vi "Digital Input 16-32.vi"(9 "S.no":string[](array[string]), 10 "Sting Array":string[](array[string]), 11 "Digital In _DAQ":bool[](array[boolean])) -> (2 "array":T1(array[cluster]))   [LabVIEW 2015]
panel:
  in  "output cluster":T2
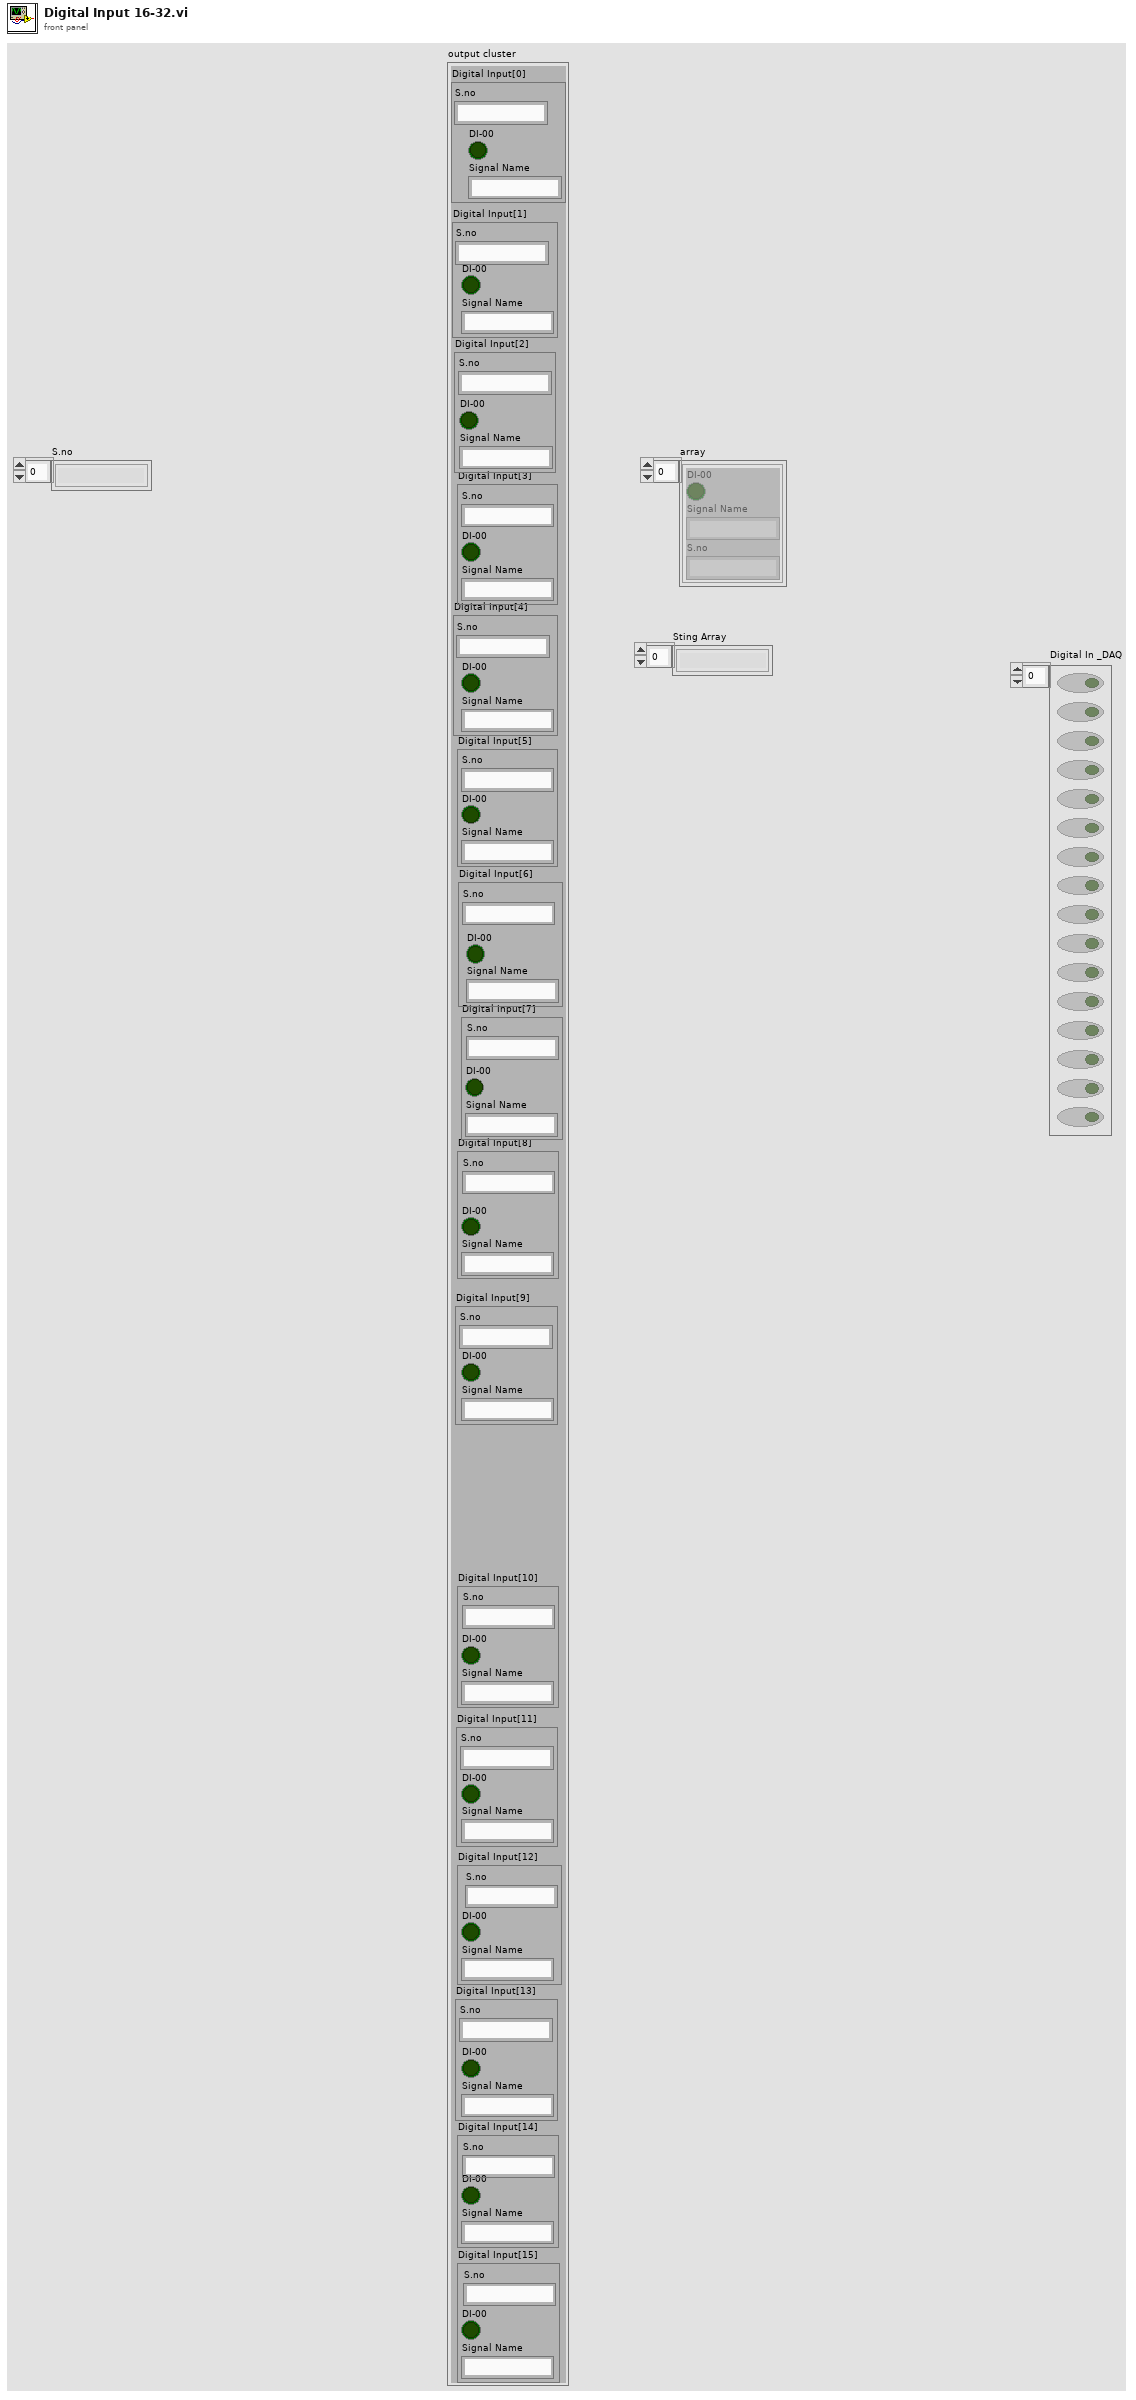
[diagram p1: front panel]
types:
  T1 = cluster{"DI-00":bool, "Signal Name":string, "S.no":string}[]
  T2 = cluster{"Digital Input[0]":cluster{"DI-00":bool, "Signal Name":string, "S.no":string}, "Digital Input[1]":cluster{"DI-00":bool, "Signal Name":string, "S.no":string}, "Digital Input[2]":cluster{"DI-00":bool, "Signal Name":string, "S.no":string}, "Digital Input[3]":cluster{"DI-00":bool, "Signal Name":string, "S.no":string}, "Digital Input[4]":cluster{"DI-00":bool, "Signal Name":string, "S.no":string}, "Digital Input[5]":cluster{"DI-00":bool, "Signal Name":string, "S.no":string}, "Digital Input[6]":cluster{"DI-00":bool, "Signal Name":string, "S.no":string}, "Digital Input[7]":cluster{"DI-00":bool, "Signal Name":string, "S.no":string}, "Digital Input[8]":cluster{"DI-00":bool, "Signal Name":string, "S.no":string}, "Digital Input[9]":cluster{"DI-00":bool, "Signal Name":string, "S.no":string}, "Digital Input[10]":cluster{"DI-00":bool, "Signal Name":string, "S.no":string}, "Digital Input[11]":cluster{"DI-00":bool, "Signal Name":string, "S.no":string}, "Digital Input[12]":cluster{"DI-00":bool, "Signal Name":string, "S.no":string}, "Digital Input[13]":cluster{"DI-00":bool, "Signal Name":string, "S.no":string}, "Digital Input[14]":cluster{"DI-00":bool, "Signal Name":string, "S.no":string}, "Digital Input[15]":cluster{"DI-00":bool, "Signal Name":string, "S.no":string}}
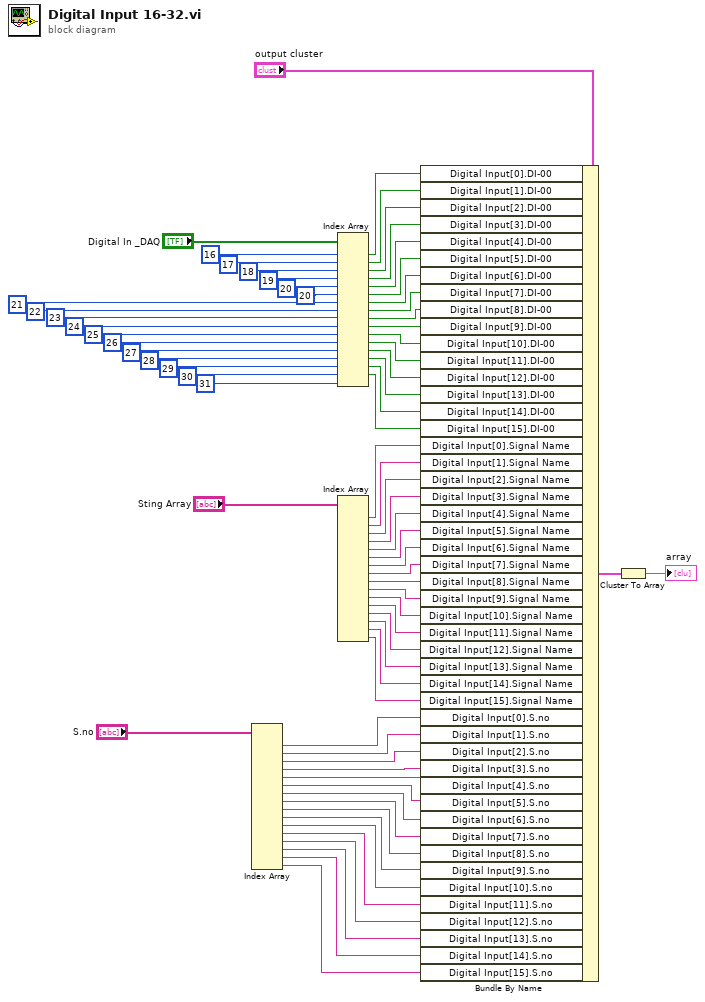
[diagram p0: block diagram]
diagram:
  n1 = Index Array(array="S.no") -> (element #1=w34:string, element #2=w32:string, element #3=w31:string, element #4=w30:string, element #5=w29:string, element #6=w28:string, element #7=w27:string, element #8=w26:string, element #9=w25:string, element #10=w24:string, element #11=w23:string, element #12=w22:string, element #13=w21:string, element #14=w20:string, element #15=w19:string, element #16=w18:string)  [unwired: 16 in]
  n2 = Index Array(array="Digital In _DAQ", index #1=16 ("index"), index #2=17 ("index"), index #3=18 ("index"), index #4=19 ("index"), index #5=20 ("index"), index #6=20 ("index"), index #7=21 ("index"), index #8=22 ("index"), index #9=23 ("index"), index #10=24 ("index"), index #11=25 ("index"), index #12=26 ("index"), index #13=27 ("index"), index #14=28 ("index"), index #15=29 ("index"), index #16=30 ("index"), index #17=31 ("index")) -> (element #1=w71:bool, element #2=w70:bool, element #3=w69:bool, element #4=w68:bool, element #5=w67:bool, element #6=w66:bool, element #7=w65:bool, element #8=w64:bool, element #9=w63:bool, element #10=w62:bool, element #11=w61:bool, element #12=w60:bool, element #13=w59:bool, element #14=w58:bool, element #15=w57:bool, element #16=w56:bool)  [unwired: 1 out]
  n3 = Index Array(array="Sting Array") -> (element #1=w54:string, element #2=w53:string, element #3=w52:string, element #4=w51:string, element #5=w50:string, element #6=w49:string, element #7=w48:string, element #8=w47:string, element #9=w46:string, element #10=w45:string, element #11=w44:string, element #12=w43:string, element #13=w42:string, element #14=w41:string, element #15=w40:string, element #16=w39:string)  [unwired: 16 in]
  n4 = Bundle By Name(cluster="output cluster", "Digital Input[0].DI-00"=w71, "Digital Input[1].DI-00"=w70, "Digital Input[2].DI-00"=w69, "Digital Input[3].DI-00"=w68, "Digital Input[4].DI-00"=w67, "Digital Input[5].DI-00"=w66, "Digital Input[6].DI-00"=w65, "Digital Input[7].DI-00"=w64, "Digital Input[8].DI-00"=w63, "Digital Input[9].DI-00"=w62, "Digital Input[10].DI-00"=w61, "Digital Input[11].DI-00"=w60, "Digital Input[12].DI-00"=w59, "Digital Input[13].DI-00"=w58, "Digital Input[14].DI-00"=w57, "Digital Input[15].DI-00"=w56, "Digital Input[0].Signal Name"=w54, "Digital Input[1].Signal Name"=w53, "Digital Input[2].Signal Name"=w52, "Digital Input[3].Signal Name"=w51, "Digital Input[4].Signal Name"=w50, "Digital Input[5].Signal Name"=w49, "Digital Input[6].Signal Name"=w48, "Digital Input[7].Signal Name"=w47, "Digital Input[8].Signal Name"=w46, "Digital Input[9].Signal Name"=w45, "Digital Input[10].Signal Name"=w44, "Digital Input[11].Signal Name"=w43, "Digital Input[12].Signal Name"=w42, "Digital Input[13].Signal Name"=w41, "Digital Input[14].Signal Name"=w40, "Digital Input[15].Signal Name"=w39, "Digital Input[0].S.no"=w34, "Digital Input[1].S.no"=w32, "Digital Input[2].S.no"=w31, "Digital Input[3].S.no"=w30, "Digital Input[4].S.no"=w29, "Digital Input[5].S.no"=w28, "Digital Input[6].S.no"=w27, "Digital Input[7].S.no"=w26, "Digital Input[8].S.no"=w25, "Digital Input[9].S.no"=w24, "Digital Input[10].S.no"=w23, "Digital Input[11].S.no"=w22, "Digital Input[12].S.no"=w21, "Digital Input[13].S.no"=w20, "Digital Input[14].S.no"=w19, "Digital Input[15].S.no"=w18) -> (w55:T2)
  n5 = Cluster To Array(cluster=w55) -> (array=→"array":T1)
